vi "Wczytanie_ustawien_AI.vi"(8 "error in (no error)":errorcluster, 10 "AI referencje Array":refnum<vi>[](array[refnum]), 11 "Plik konf in":path=path "D:/Marek/Dysk Google/Projekty LabVIEW/! Rudpol/Program/Konfiguracja/AI_Konfiguracja.txt") -> (0 "error out":errorcluster, 2 "AiParamsOut":T1[](array[typedef]) {"Numer" min=1 max=8 step=1}, 3 "Plik konf out":path)   [LabVIEW 2013]
doc: "Use this template to build a VI to use as a subVI."
uses:
  Kontrolki/GUI/AI_parametry.ctl
  Kontrolki/GUI/AI_wartosc.ctl
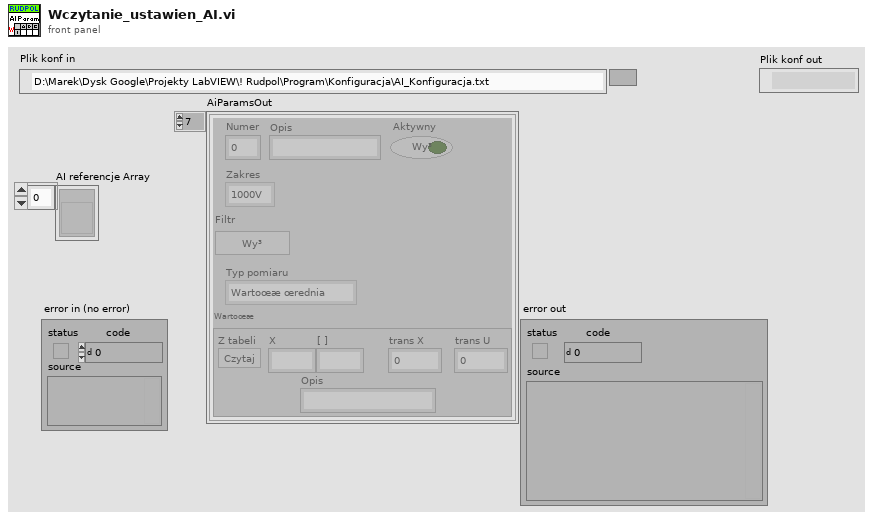
[diagram p1: front panel]
types:
  T1 = typedef "AI_parametry.ctl" = cluster{"Numer":u8, "Opis":string, "Zakres":enum16{"1000V", "300V", "30V", "3V", "0,3V"}, "Filtr":bool, "Typ pomiaru":enum16{"Wartoœæ œrednia", "Œrednia wyprostowana", "Wartoœæ skuteczna"}, "Aktywny":bool, "Wartoœæ":T2}
  T2 = typedef "AI_wartosc.ctl" = cluster{"X":string, "[ ]":string, "trans X":dbl, "trans U":dbl, "Z tabeli":bool, "Opis":string}
  T3 = enum16{"open", "replace", "create", "open or create", "replace or create", "replace or create with confirmation"}
  T4 = enum16{"Wartoœæ œrednia", "Œrednia wyprostowana", "Wartoœæ skuteczna"}
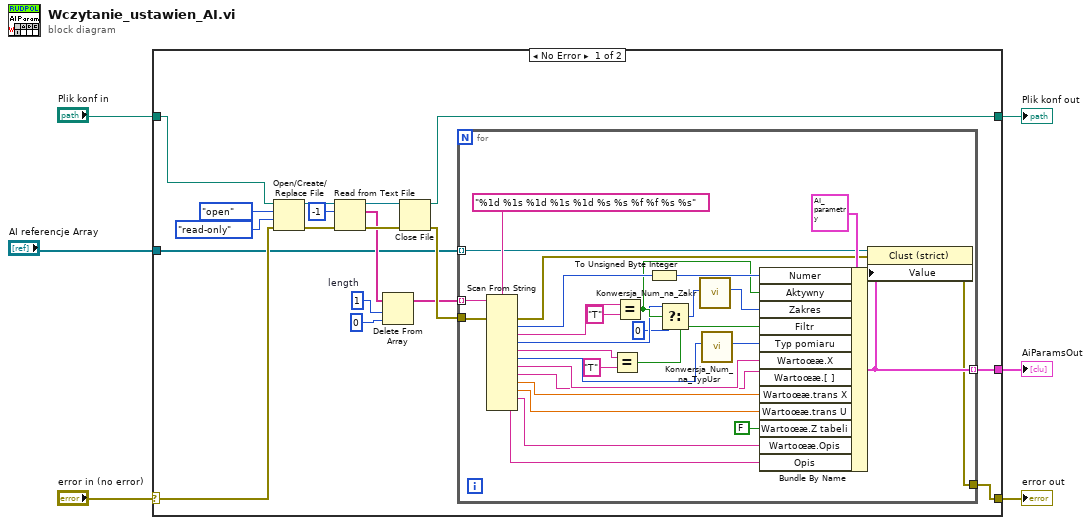
[diagram p0: block diagram]
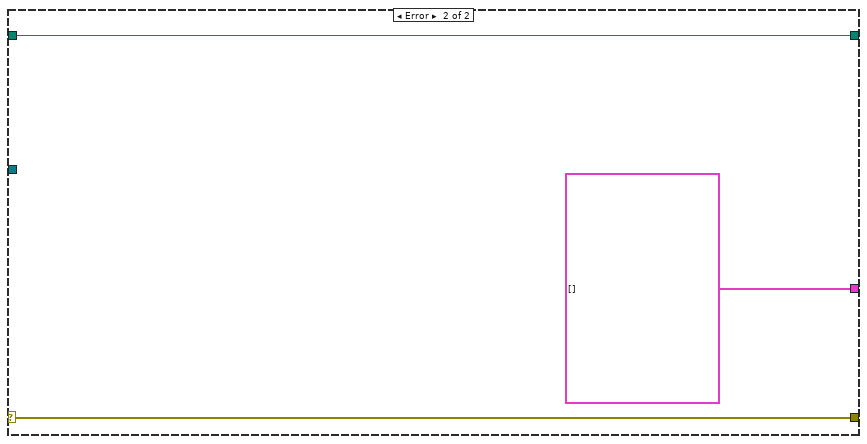
[diagram p2: hidden frame]
diagram:
  n1 = case shown="No Error" "error in (no error)" {
    selector: "error in (no error)" -> [w12 w56]
    tunnel: [w11 w56] -> w5
    tunnel: "Plik konf in" -> [w17 w55]
    tunnel: [w16 w55] -> w4
    tunnel: [w10 T1[] []] -> w3
    tunnel: "AI referencje Array" -> [w7 _]
    frame No Error {
      w14 = 1  # length
      n2 = Open/Create/Replace File(file path (use dialog)=w17, error in=w12, operation (0:open)=T3."open", access (0:read/write)=enum16{"read/write", "read-only", "write-only"}."read-only") -> (refnum out=w21:refnum<file>, error out=w22:errorcluster)  [unwired: 2 in, 1 out]
      n3 = Read from Text File(file (use dialog)=w21, count=-1, error in=w22) -> (refnum out=w19:refnum<file>, text=w9:string[], error out=w20:errorcluster)  [unwired: 1 in, 1 out]
      n4 = Delete From Array(array=w9, length=w14, index=0) -> (array with subset deleted=w8:string[])  [unwired: 1 out]
      n5 = Close File(refnum=w19, error in=w20) -> (path=w16:path, error out=w13:errorcluster)
      n6 = for {
        tunnel: w8 -> [w52] mode=indexing
        tunnel: w13 -> [w51]
        tunnel: [w29] -> w11
        tunnel: [w31] -> w10 mode=indexing
        tunnel: w7 -> [w32] mode=indexing
        n7 = Scan From String(format string="%1d %1s %1d %1s %1d %s %s %f %f %s %s", input string=w52, error in=w51) -> (error out=w30:errorcluster, output 1=w48:i32, output 2=w45:string, output 3=w27:i32, output 4=w40:string, output 5=w39:i32, output 6=w38:string, output 7=w37:string, output 8=w36:dbl, output 9=w35:dbl, output 10=w34:string, output 11=w33:string)  [unwired: 12 in, 2 out]
        n8 = Equal?(x=w40, y="T") -> (x = y?=w42:bool)
        n9 = Equal?(x=w45, y="T") -> (x = y?=w28:bool)
        n10 = To Unsigned Byte Integer(number=w48) -> (unsigned 8bit integer=w50:u8)
        n11 = Select(t=w27, s=w28, f=0) -> (s? t:f=w26:i32)
        n12 = call "Konwersja_Num_na_Zakr.vi"("Zakres No"=w26) -> ("Zakres out"=w44:enum16{"1000V", "300V", "30V", "3V", "0,3V"})  [unwired: 10 in]
        n13 = call "Konwersja_Num_na_TypUsr.vi"("Zakres No"=w39) -> ("Typ pomiaru"=w43:T4)  [unwired: 10 in]
        n14 = Bundle By Name(cluster=T1 {"Numer"=1, "Opis"="Kana³ 1", "Zakres"=enum."1000V", "Filtr"=FALSE, "Typ pomiaru"=enum."Wartoœæ œrednia", "Aktywny"=FALSE, "Wartoœæ"={"X"="U", "[ ]"="V", "trans X"=1.0, "trans U"=1.0, "Z tabeli"=FALSE, "Opis"=""}} ("AI_parametry"), "Numer"=w50, "Aktywny"=w28, "Zakres"=w44, "Filtr"=w42, "Typ pomiaru"=w43, "Wartoœæ.X"=w38, "Wartoœæ.[ ]"=w37, "Wartoœæ.trans X"=w36, "Wartoœæ.trans U"=w35, "Wartoœæ.Z tabeli"=FALSE, "Wartoœæ.Opis"=w34, "Opis"=w33) -> (w31:T1)
        n15 = property class="Clust (strict)"(reference=w32, error in=w30, "Value"=w31) -> (error out=w29:errorcluster)  [unwired: 1 out]
      }
    }
    frame Error {
    }
  }
  "error out" <- w5
  "Plik konf out" <- w4
  "AiParamsOut" <- w3
